vi "pump rpm all tubing.vi"(0 "Pump":T2 {"0 to 1" format="%.2f"; "flow rate" format="%.2f"}, 1 "pump ID":u8) -> (3 "pump speed (%)":dbl format="%.2f", 4 "pump volts (0-5)":dbl format="%.2f", 5 "Pump dir on":T1[](array[typedef]))   [LabVIEW 2015]
uses:
  Peristaltic/Pump w direction.ctl
  mini peristaltic pump.ctl
  Pump Direction.ctl
  3-stop colors and numbers.ctl
  calibration commands.ctl
panel:
  out "STAMP slope out":dbl=2.52
  out "STAMP intercept out":dbl
  in  "mL per rev":sgl[](array[numeric])=[0.001518497, 0.003209591, 0.005497798, 0.012406906, 0.016451517, 0.021816157, 0.026944764, 0.03351825, 0.04617598, 0.061704744, 0.069453366, 0.0789204, 0.088816434, 0.09612975, 0.10822253, 0.12075485, 0.14027181, 0.15709075, 0.17954482, 0.19715126, 0.2149444, 0.252498, 0.29306096, 0.3351765, 0.37380016, 0.42250744, 0.06, 0.21, 1.7, 0.8, 2.8, 3.8] format="%.7f"
  in  "IDs":sgl[](array[numeric])=[0.13, 0.19, 0.25, 0.38, 0.44, 0.51, 0.57, 0.64, 0.76, 0.89, 0.95, 1.02, 1.09, 1.14, 1.22, 1.3, 1.42, 1.52, 1.65, 1.75, 1.85, 2.06, 2.29, 2.54, 2.79, 3.17, 0.79375, 1.5875, 4.8, 3.175, 6.35, 7.9375] format="%.3f"
  # "orange-black\norange-red\norange-blue\norange-green\ngreen-yellow\norange-yellow\nwhite-yellow\norange-white\nblack-black\norange-orange\nwhite-black\nwhite-white\nwhite-red\nred-red\nred-grey\ngrey-grey\nyellow-yellow\nyellow-blue\nblue-blue\nblue-green\ngreen-green\npurple-purple\npurple-black\npurple-orange\npurple-white\nblack-white\n13\n14\n15\n16\n17\n18"
  # "13"
  # "14"
  # "15"
  # "16"
  # "17"
  # "18"
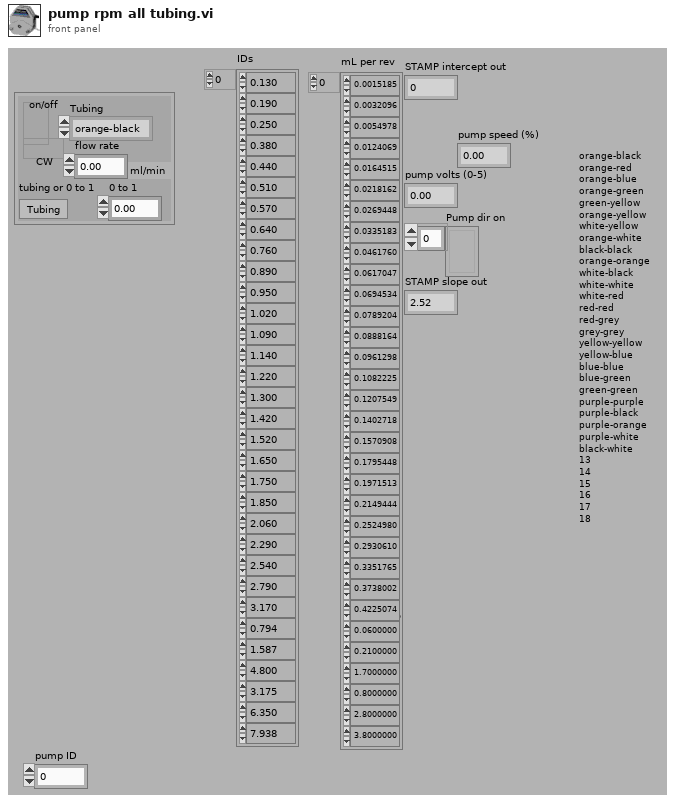
[diagram p1: front panel]
types:
  T1 = typedef "mini peristaltic pump.ctl" = bool
  T2 = typedef "Pump w direction.ctl" = cluster{"on/off":T1, "Direction":T3, "flow rate":dbl[unit], "Tubing":T4, "tubing or 0 to 1":bool, "0 to 1":dbl}
  T3 = typedef "Pump Direction.ctl" = bool
  T4 = typedef "3-stop colors and numbers.ctl" = enum16{"orange-black", "orange-red", "orange-blue", "orange-green", "green-yellow", "orange-yellow", "white-yellow", "orange-white", "black-black", "orange-orange", "white-black", "white-white", "white-red", "red-red", "red-grey", "grey-grey", "yellow-yellow", "yellow-blue", "blue-blue", "blue-green", "green-green", "purple-purple", "purple-black", "purple-orange", "purple-white", "black-white", "13", "14", "15", "16", "17", "18"}
  T5 = typedef "calibration commands.ctl" = enum16{"Get ini Path", "Save default values", "Save new calibration", "Read calibration", "Apply calibration", "Read STAMP mb", "Write STAMP mb"}
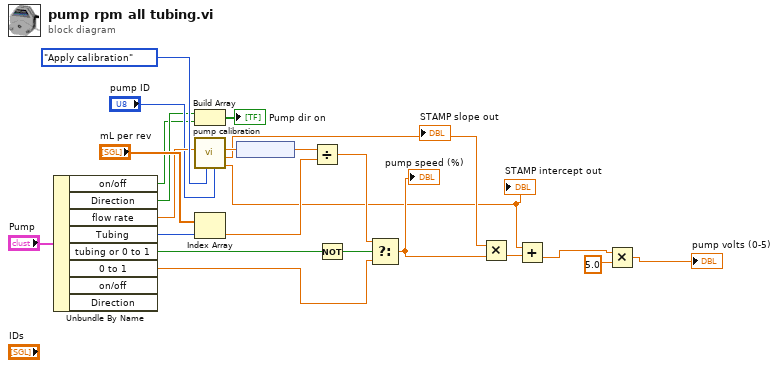
[diagram p0: block diagram]
diagram:
  n1 = Unbundle By Name("Pump") -> ("on/off"=w9:T1, "Direction"=w10:T3, "flow rate"=w18:dbl[unit], "Tubing"=w17:T4, "tubing or 0 to 1"=w16:bool, "0 to 1"=w2:dbl)  [unwired: 2 out]
  n2 = Build Array(w10, w9) -> (→"Pump dir on":T1[])
  n3 = call "pump calibration.vi"("pump ID"="pump ID", "pump cal command"=calibration_commands."Apply calibration", "flow rate"=w18) -> ("STAMP intercept out"=w1:dbl, "STAMP slope out"=w6:dbl, "modified flow rate"=w21:dbl[unit])  [unwired: 5 in, 1 out]
  "STAMP intercept out" <- w1
  "STAMP slope out" <- w6
  n4 = Index Array(array="mL per rev", index=w17) -> (element=w20:sgl)
  n5 = node(w21) -> (w23:dbl)
  n6 = Divide(x=w23, y=w20) -> (x/y=w15:dbl)
  n7 = Not(x=w16) -> (.not. x?=w14:bool)
  n8 = Select(t=w15, s=w14, f=w2) -> (s? t:f=w5:dbl)
  "pump speed (%)" <- w5
  n9 = Multiply(x=w6, y=w5) -> (x*y=w7:dbl)
  n10 = Add(x=w1, y=w7) -> (x+y=w4:dbl)
  n11 = Multiply(x=w4, y=5.0) -> (x*y=→"pump volts (0-5)":dbl)
